vi "rpc_tsmaster_is_simulation_running.vi"(8 "error in (no error)":errorcluster caption="错误输入（无错误）", 9 "AHandle":u32, 11 "路径输入":path) -> (0 "error out":errorcluster caption="错误输出", 1 "AIsRunning":bool, 2 "function return":i32, 3 "路径输出":path)   [LabVIEW 2014]
doc: "Function introduction: Obtain the status of remote TSMaster simulation operation\nAfter calling the location to create TSMaster Rpc client\nInput parameter AHHandle: TSMaster Rpc client handle\nAIsRunning: Data pointer for the status of remote TSMaster simulation running\nTrue=Running, false=Not Running\nReturn value==0: Function execution successful\nOther values: Function execution failed"
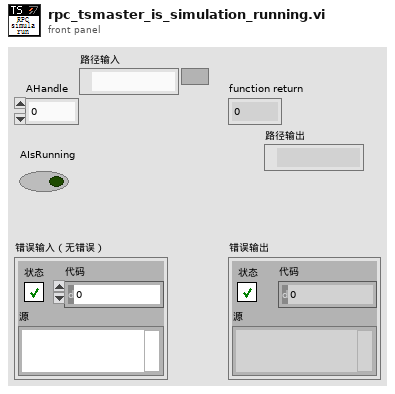
[diagram p1: front panel]
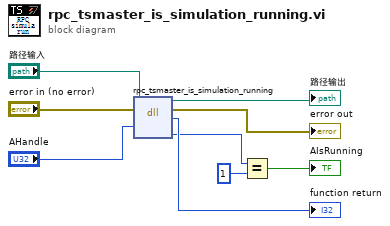
[diagram p0: block diagram]
diagram:
  n1 = dll-call lib="D:/Work/LabVIEW Code/TSMaster Labview SDK/LabVIEW/LabVIEW-TSMasterAPI_CLN/TSMasterAPI_LabVIEW-2024-10-08 14-20-13/Not_organized_vi/TSMaster.*" fn="rpc_tsmaster_is_simulation_running"(path in="路径输入", error in="error in (no error)", "AHandle"="AHandle") -> (path out=→"路径输出":path, error out=→"error out":errorcluster, "返回类型"=→"function return":i32, "AIsRunning"=w3:u8)  [unwired: 3 in]
  n2 = Equal?(x=w3, y=u8 1) -> (x = y?=→"AIsRunning":bool)
